vi "Log Error.vi"(8 "error in (no error)":errorcluster, 11 "Da Base in":refnum<class "Application Controller.lvclass">) -> (0 "error out":errorcluster, 1 "Error message":string, 2 "stop actor?":bool=TRUE, 3 "Da Base out":refnum<class "Application Controller.lvclass">, 4 "LabActor Error":T1)   [LabVIEW 2019, in "Application Controller.lvclass"]
uses:
  Application Controller.lvclass
  <vilib>/Utility/error.llb/Error Cluster From Error Code.vi
  <vilib>/ErrorRing/Error Ring.xnode
  <vilib>/Utility/sysdir.llb/System Directory Type.ctl
  <vilib>/Utility/error.llb/DialogType.ctl
  Template Module/LabActor Error.ctl
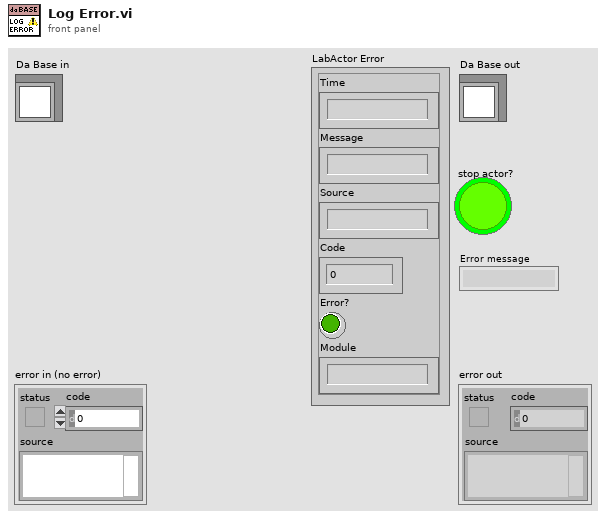
[diagram p1: front panel]
types:
  T1 = typedef "LabActor Error.ctl" = cluster{"Time":string, "Message":string, "Source":string, "Code":i32, "Error?":bool, "Module":string}
  T2 = enum16{"open", "replace", "create", "open or create", "replace or create", "replace or create with confirmation"}
  T3 = typedef "DialogType.ctl" = u16
  T4 = typedef "System Directory Type.ctl" = i32
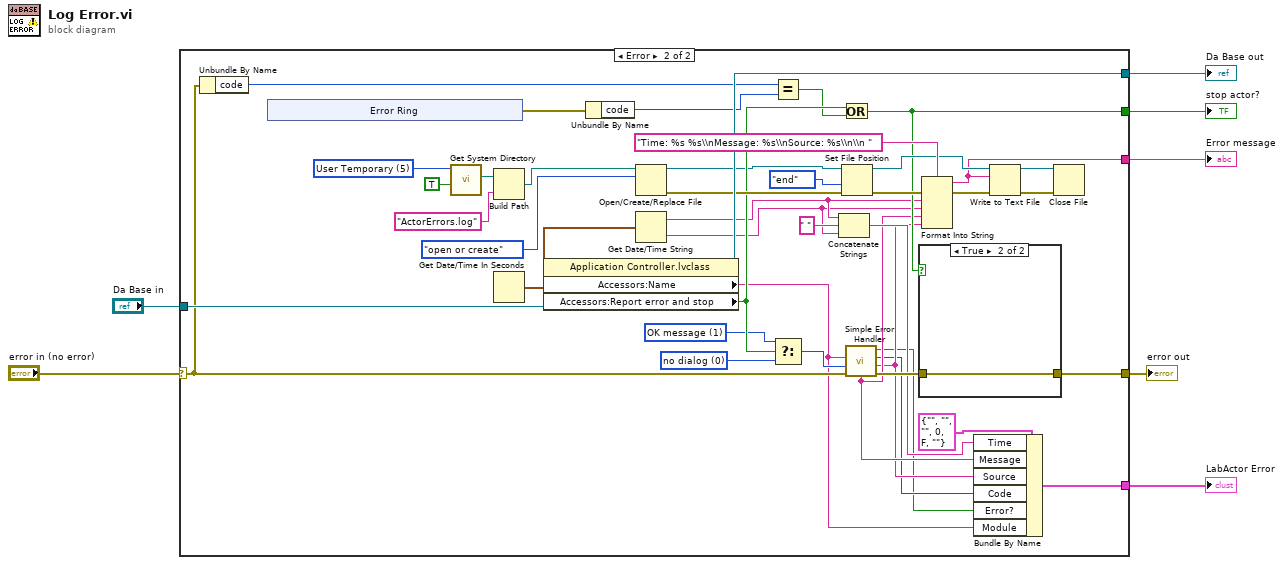
[diagram p0: block diagram]
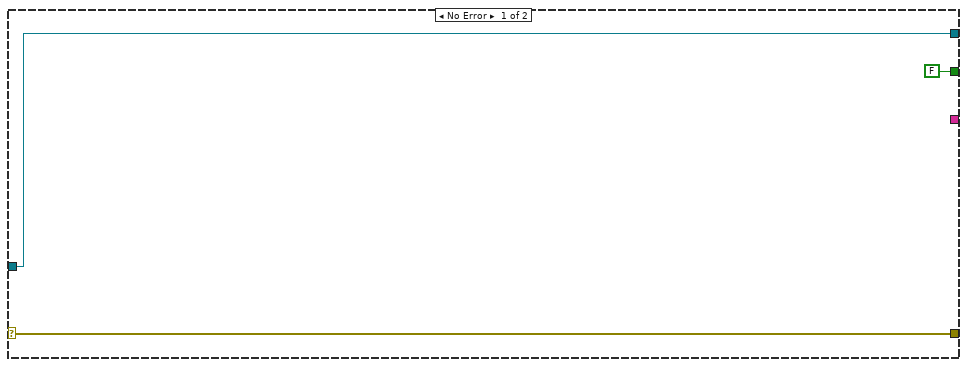
[diagram p2: hidden frame]
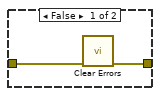
[diagram p3: hidden frame]
diagram:
  n1 = case shown="Error" "error in (no error)" {
    selector: "error in (no error)" -> [w9 w49]
    tunnel: [w9 w33] -> w6
    tunnel: [w10 w51] -> w4
    tunnel: "Da Base in" -> [w10 w52]
    tunnel: [FALSE ("Accessors:Report error and stop") w23] -> w3
    tunnel: [_ w27] -> w2
    tunnel: [_ w16] -> w1
    frame No Error {
    }
    frame Error {
      w25 = T3 1 items=["no dialog", "OK message", "continue or stop message", "OK message + warnings", "continue/stop + warnings"] ("type of dialog (OK msg:1)")
      w26 = T3 0 items=["no dialog", "OK message", "continue or stop message", "OK message + warnings", "continue/stop + warnings"] ("type of dialog (OK msg:1)")
      w46 = T4 5 items=["User Home"=0, "User Desktop"=1, "User Documents"=2, "User Application Data"=3, "User Preferences"=4, "User Temporary"=5, "Public Documents"=6, "Public Application Data"=7, "Public Preferences"=8, "Public Cache"=13, "System Core Libraries"=9, "System Installed Libraries"=10, "Application Files"=11, "Boot Volume Root"=12] ("system directory type")
      n2 = Unbundle By Name(w49) -> ("code"=w48:i32)
      n3 = xnode "Error Ring"() -> ("error out"=w50:errorcluster)
      n4 = call <vilib>:"Get System Directory.vi"("create directory if not found? (F)"=TRUE, "system directory type"=w46) -> ("system directory"=w44:path)  [unwired: 9 in]
      n5 = Build Path(base path=w44, name or relative path="ActorErrors.log") -> (appended path=w42:path)
      n6 = Get Date/Time In Seconds() -> (seconds since 1Jan1904=w39:timestamp)
      n7 = property class="Application Controller.lvclass"(reference=w52) -> (reference out=w51:refnum<class "Application Controller.lvclass">, "Accessors:Name"=w11:string, "Accessors:Report error and stop"=w32:bool)  [unwired: 1 in, 1 out]
      n8 = Unbundle By Name(w50) -> ("code"=w47:i32)
      n9 = Open/Create/Replace File(file path (use dialog)=w42, operation (0:open)=T2."open or create") -> (refnum out=w30:refnum<file>, error out=w38:errorcluster)  [unwired: 4 in, 1 out]
      n10 = Get Date/Time String(seconds (now)=w39) -> (date string=w19:string, time string=w17:string)  [unwired: 2 in]
      n11 = Equal?(x=w48, y=w47) -> (x = y?=w22:bool)
      n12 = Select(t=w25, s=w32, f=w26) -> (s? t:f=w24:T3)
      n13 = Concatenate Strings(w19, " " ("string"), w17) -> (w20:string)
      n14 = Or(x=w32, y=w22) -> (x .or. y?=w23:bool)
      n15 = Set File Position(refnum=w30, from (0:start)=enum16{"start", "end", "current"}."end", error in=w38) -> (refnum out=w29:refnum<file>, error out=w31:errorcluster)  [unwired: 1 in]
      n16 = call <vilib>:"Simple Error Handler.vi"("error source (\" \")"=w11, "type of dialog (OK msg:1)"=w24, "error in (no error)"=w49) -> ("error?"=w12:bool, "code out"=w13:i32, "source out"=w14:string, "error out"=w34:errorcluster, "message"=w15:string)  [unwired: 2 in]
      n17 = case shown="True" w23 {
        tunnel: w34 -> [w54 w55]
        tunnel: [w53 w55] -> w33
        frame False {
          n18 = call <vilib>:"Clear Errors.vi"("error in (no error)"=w54) -> ("error out"=w53:errorcluster)  [unwired: 5 in, 1 out]
        }
        frame True {
        }
      }
      n19 = Format Into String(format string="Time: %s %s\\nMessage: %s\\nSource: %s\\n\\n ", error in=w31, w19, w17, w15, w14) -> (resulting string=w27:string, error out=w37:errorcluster)  [unwired: 1 in]
      n20 = Bundle By Name(cluster=T1 {"Time"="", "Message"="", "Source"="", "Code"=0, "Error?"=FALSE, "Module"=""} ("LabActor Error"), "Time"=w20, "Message"=w15, "Source"=w14, "Code"=w13, "Error?"=w12, "Module"=w11) -> (w16:T1)
      n21 = Write to Text File(file (use dialog)=w29, text=w27, error in=w37) -> (refnum out=w36:refnum<file>, error out=w35:errorcluster)  [unwired: 1 in, 1 out]
      n22 = Close File(refnum=w36, error in=w35) -> ()  [unwired: 2 out]
    }
  }
  "error out" <- w6
  "Da Base out" <- w4
  "stop actor?" <- w3
  "Error message" <- w2
  "LabActor Error" <- w1
